vi "Auto-Register For Events.vi"(7 "Use Label Text (F=Use Caption)":bool, 8 "error in (no error)":errorcluster, 9 "Controls to Exclude":refnum<vi>[](array[refnum]), 10 "VI Refnum (Actor Core)":refnum<vi>, 11 "EventAggregator Enqueuer":refnum<class "Message Enqueuer.lvclass">) -> (0 "error out":errorcluster, 3 "ActorAutoRegistration Out":refnum<class "ActorAutoRegistration.lvclass">)   [LabVIEW 2015, in "ActorEvents.lvlib" / "ActorAutoRegistration.lvclass"]
doc: "<License>\nCopyright © 2017 Composed Systems, LLC | All rights reserved\nwww.composed.io\n\nAuthor: Ethan Stern <ethan.stern@composed.io>\n\nThis software is provided \"AS IS\" WITHOUT WARRANTIES, either express or implied, AND IS FOR EDUCATIONAL PURPOSES ONLY.\n</License>"
uses:
  ActorAutoRegistration.lvclass
  <vilib>/ActorFramework/Message Enqueuer/Message Enqueuer.lvclass
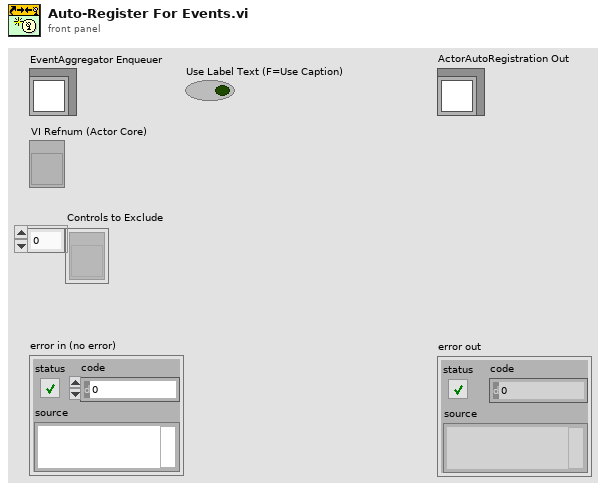
[diagram p1: front panel]
types:
  T1 = cluster{"ClassName":string, "Control Refnums":refnum<vi>[]}[]
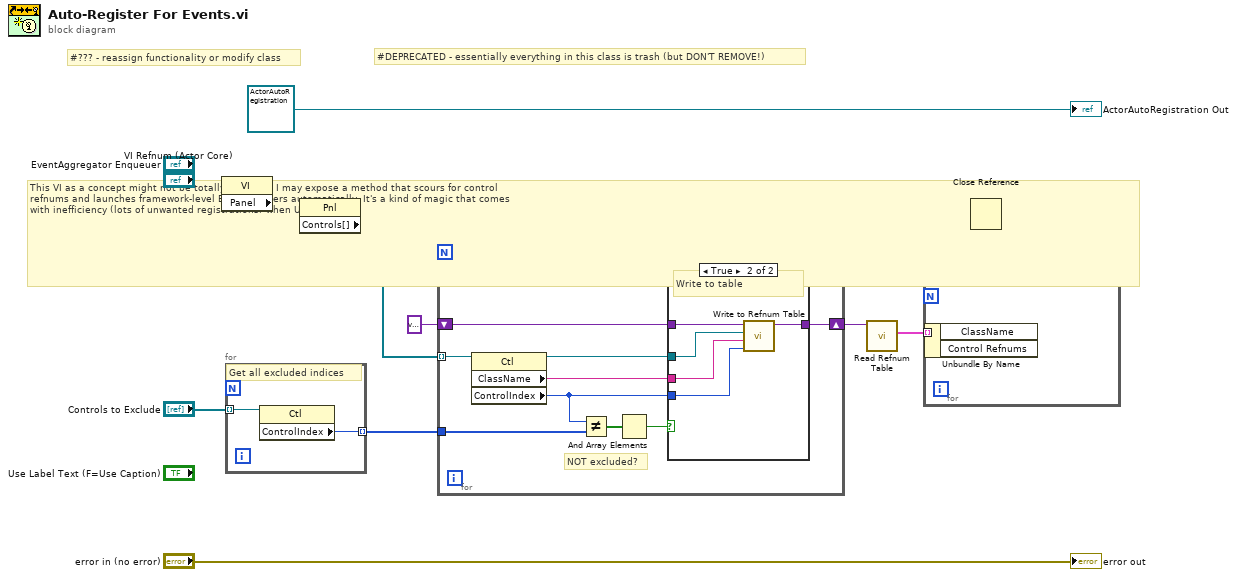
[diagram p0: block diagram]
diagram:
  # "This VI as a concept might not be totally useless -- I may expose a method that scours for control\nrefnums and launches framework-level EventHandlers automatically. It's a kind of magic that comes\nwith inefficiency (lots of unwanted registrations) when UIs get large."
  # "#DEPRECATED - essentially everything in this class is trash (but DON'T REMOVE!)"
  # "#??? - reassign functionality or modify class"
  n1 = property class="VI"(reference="VI Refnum (Actor Core)") -> ("Panel"=w8:refnum<vi>)  [unwired: 1 in, 2 out]
  n2 = for {
    tunnel: "Controls to Exclude" -> [w13] mode=indexing
    tunnel: [w12] -> w5 mode=indexing
    # "Get all excluded indices"
    n3 = property class="Ctl"(reference=w13) -> ("ControlIndex"=w12:i32)  [unwired: 1 in, 2 out]
  }
  n4 = property class="Pnl"(reference=w8) -> (reference out=w4:refnum<vi>, "Controls[]"=w7:refnum<vi>[])  [unwired: 1 in, 1 out]
  n5 = for {
    tunnel: w7 -> [w22] mode=indexing
    tunnel: w5 -> [w21]
    shift-right: [w18] -> w2
    shift-left: variant -> [w17]
    # "NOT excluded?"
    n6 = property class="Ctl"(reference=w22) -> (reference out=w15:refnum<vi>, "ClassName"=w19:string, "ControlIndex"=w16:i32)  [unwired: 1 in, 1 out]
    n7 = Not Equal?(x=w16, y=w21) -> (x != y?=w20:bool[])
    n8 = And Array Elements(Boolean array=w20) -> (logical AND=w14:bool)
    n9 = case shown="True" w14 {
      tunnel: w19 -> [_ w28]
      tunnel: [w23 w27] -> w18
      tunnel: w17 -> [w23 w26]
      tunnel: w16 -> [_ w25]
      tunnel: w15 -> [_ w24]
      frame False {
        # "Do not write"
      }
      frame True {
        # "Write to table"
        n10 = call "Write to Refnum Table.vi"("ControlIndex"=w25, "ClassName"=w28, "Control Refnum"=w24, "Typed Refnum Table In"=w26) -> ("Typed Refnum Table Out"=w27:variant)  [unwired: 7 in]
      }
    }
  }
  n11 = call "Read Refnum Table.vi"("Typed Refnum Table In"=w2) -> ("Refnum Groups"=w1:T1)  [unwired: 10 in]
  n12 = for {
    tunnel: w1 -> [w29] mode=indexing
    n13 = Unbundle By Name(w29) -> ()  [unwired: 2 out]
  }
  n14 = Close Reference(reference=w4) -> ()  [unwired: 1 in, 1 out]
  "ActorAutoRegistration Out" <- refnum<class "ActorAutoRegistration.lvclass"> refnum ("AbstractAutoRegistration in")
  "error out" <- "error in (no error)"
